vi "GetDisplayRef.vi"(8 "error in":errorcluster) -> (0 "error out":errorcluster, 3 "Picture out":refnum<vi>)   [LabVIEW 2017]
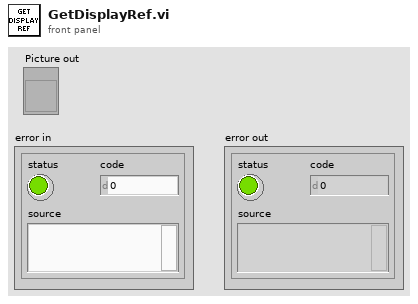
[diagram p1: front panel]
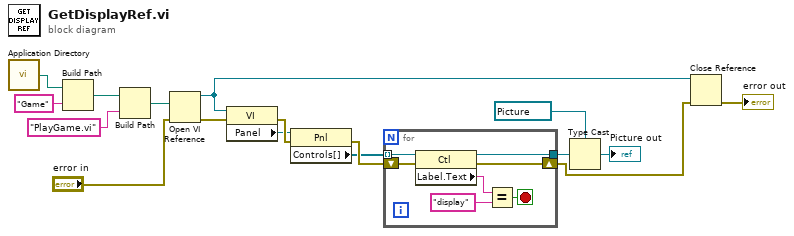
[diagram p0: block diagram]
diagram:
  n1 = call <vilib>:"Application Directory.vi"() -> ("Application Directory"=w4:path)
  n2 = Build Path(base path=w4, name or relative path="Game") -> (appended path=w6:path)
  n3 = Build Path(base path=w6, name or relative path="PlayGame.vi") -> (appended path=w8:path)
  n4 = Open VI Reference(vi path=w8, error in (no error)="error in") -> (vi reference=w3:refnum<vi>, error out=w10:errorcluster)  [unwired: 4 in]
  n5 = property class="VI"(reference=w3, error in=w10) -> (error out=w13:errorcluster, "Panel"=w11:refnum<vi>)  [unwired: 1 out]
  n6 = property class="Pnl"(reference=w11, error in=w13) -> (error out=w14:errorcluster, "Controls[]"=w12:refnum<vi>[])  [unwired: 1 out]
  n7 = for {
    tunnel: w12 -> [w24] mode=indexing
    tunnel: [w20] -> w15
    shift-right: [w18] -> w2
    shift-left: w14 -> [w19]
    stop <- w21 stop-if-true
    n8 = property class="Ctl"(reference=w24, error in=w19) -> (reference out=w20:refnum<vi>, error out=w18:errorcluster, "Label.Text"=w23:string)
    n9 = Equal?(x=w23, y="display") -> (x = y?=w21:bool)
  }
  n10 = Type Cast(type=refnum<vi> refnum ("displayRef"), x=w15) -> (*(type *) &x=→"Picture out":refnum<vi>)
  n11 = Close Reference(reference=w3, error in (no error)=w2) -> (error out=→"error out":errorcluster)
